vi "AOL Control-4ch_AC.vi"() -> ()   [LabVIEW 2020]
uses:
  TypeDef/Frequency-4ch.ctl
  TypeDef/Amplitude-4ch.ctl
  Globals/FPGA Globals.vi
  <vilib>/DAQmx/create/channels.llb/DAQmx Create Channel (CO-Pulse Generation-Time).vi
  <vilib>/FPGAPlugInAG/PXIe-7976R/niLvFpga_Open_PXIe-7976R.vi
  <vilib>/rvi/interface/common/dynamic/niFpgaDynamicAddResources.vi
  <vilib>/Utility/error.llb/Error Cluster From Error Code.vi
  <vilib>/rvi/errors/niLvFpgaAdjustHostInterfaceError.vi
  <vilib>/FPGAPlugInAG/Dynamic/niLvFpga_Close_Dynamic.vi
  <vilib>/rvi/interface/nirviOpenFPGA/nirviOpenFPGA.xnode
  FPGA Bitfiles/aolcontrolprojec_FPGATarget_Gentrigpulse_Cnv+VIMB-cw_AC.lvbitx
  <vilib>/rvi/interface/nirviReadWriteControl/nirviReadWriteControl.xnode
  <vilib>/rvi/interface/nirviCloseFPGA/nirviCloseFPGA.xnode
  NiFpgaLv.dll
  <vilib>/rvi/interface/Simulation/niFpgaSimulationCallBeginRW.vi
panel:
  in  "Tab Control":T1(tab)
  in  "Use RF from file":bool
  in  "RF Code File":path=path "D:/Microscope data/2019-04-16/Sameer/Packets"
  in  "Frequency (MHz)":T2={"Ch 1"=39, "Ch 2"=39, "Ch 3"=39, "Ch 4"=39} {"Ch 4" min=20 max=50 step=1; "Ch 3" min=20 max=50 step=1; "Ch 2" min=20 max=50 step=1; "Ch 1" min=20 max=50 step=1}
  in  "Amplitude":T3={"Ch 1"=255, "Ch 2"=255, "Ch 3"=255, "Ch 4"=255} {"Ch 4" max=255 step=1; "Ch 3" max=255 step=1; "Ch 2" max=255 step=1; "Ch 1" max=255 step=1}
  in  "Stop":bool
  in  "Load":bool
  in  "Run":bool
  in  "Clear":bool
  in  "Settings":bool
  out "Ethernet Port Opened":bool
  out "RF Loaded":bool
  out "Trigger Sent":bool
  out "Status":string
  in  "Use FlexRIO Trigger":bool=TRUE
  in  "DAQmx Trigger Channel":tag="PXI1Slot4/ctr0"
  in  "Pulse Width (sec)":dbl=1e-05
  in  "Initial Delay(sec)":dbl=0.01 format="%.6f"
  out "Select Device 1":i32=1 caption="Device 1 Port" min=1 max=5 step=1
  out "Select Device 2":i32=1 caption="Device 2 Port" min=1 max=5 step=1
  out "Packet Array":string[](array[string])
  out "No of Packets":i32
  out "FPGA MAC 1":string caption="Device 1 MAC Address"
  out "FPGA MAC 2":string caption="Device 2 MAC Address"
  out "Trigger Error":errorcluster
  in  "error in":errorcluster
  # "User needs to send a single TTL rising edge for the controller to generate RF."
  # "Trigger"
  # "Ethernet"
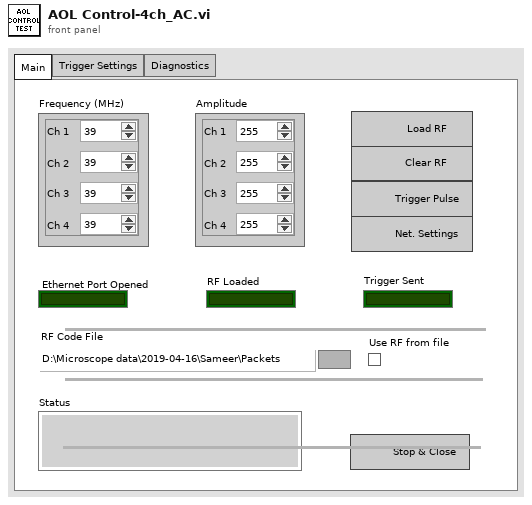
[diagram p1: front panel]
types:
  T1 = enum32{"Main", "Trigger Settings", "Diagnostics"}
  T2 = typedef "Frequency-4ch.ctl" = cluster{"Ch 1":u16, "Ch 2":u16, "Ch 3":u16, "Ch 4":u16}
  T3 = typedef "Amplitude-4ch.ctl" = cluster{"Ch 1":u16, "Ch 2":u16, "Ch 3":u16, "Ch 4":u16}
  T4 = enum8{"Enabled", "Disabled", "Disabled and Grayed Out"}
  T5 = typedef "FPGA Settings.ctl" = cluster{"System Clock(MHz)":dbl, "FPGA MAC 1":string, "Port Number 1":i32, "Port Number 2":i32, "FPGA MAC 2":string, "PC MAC Address":string}
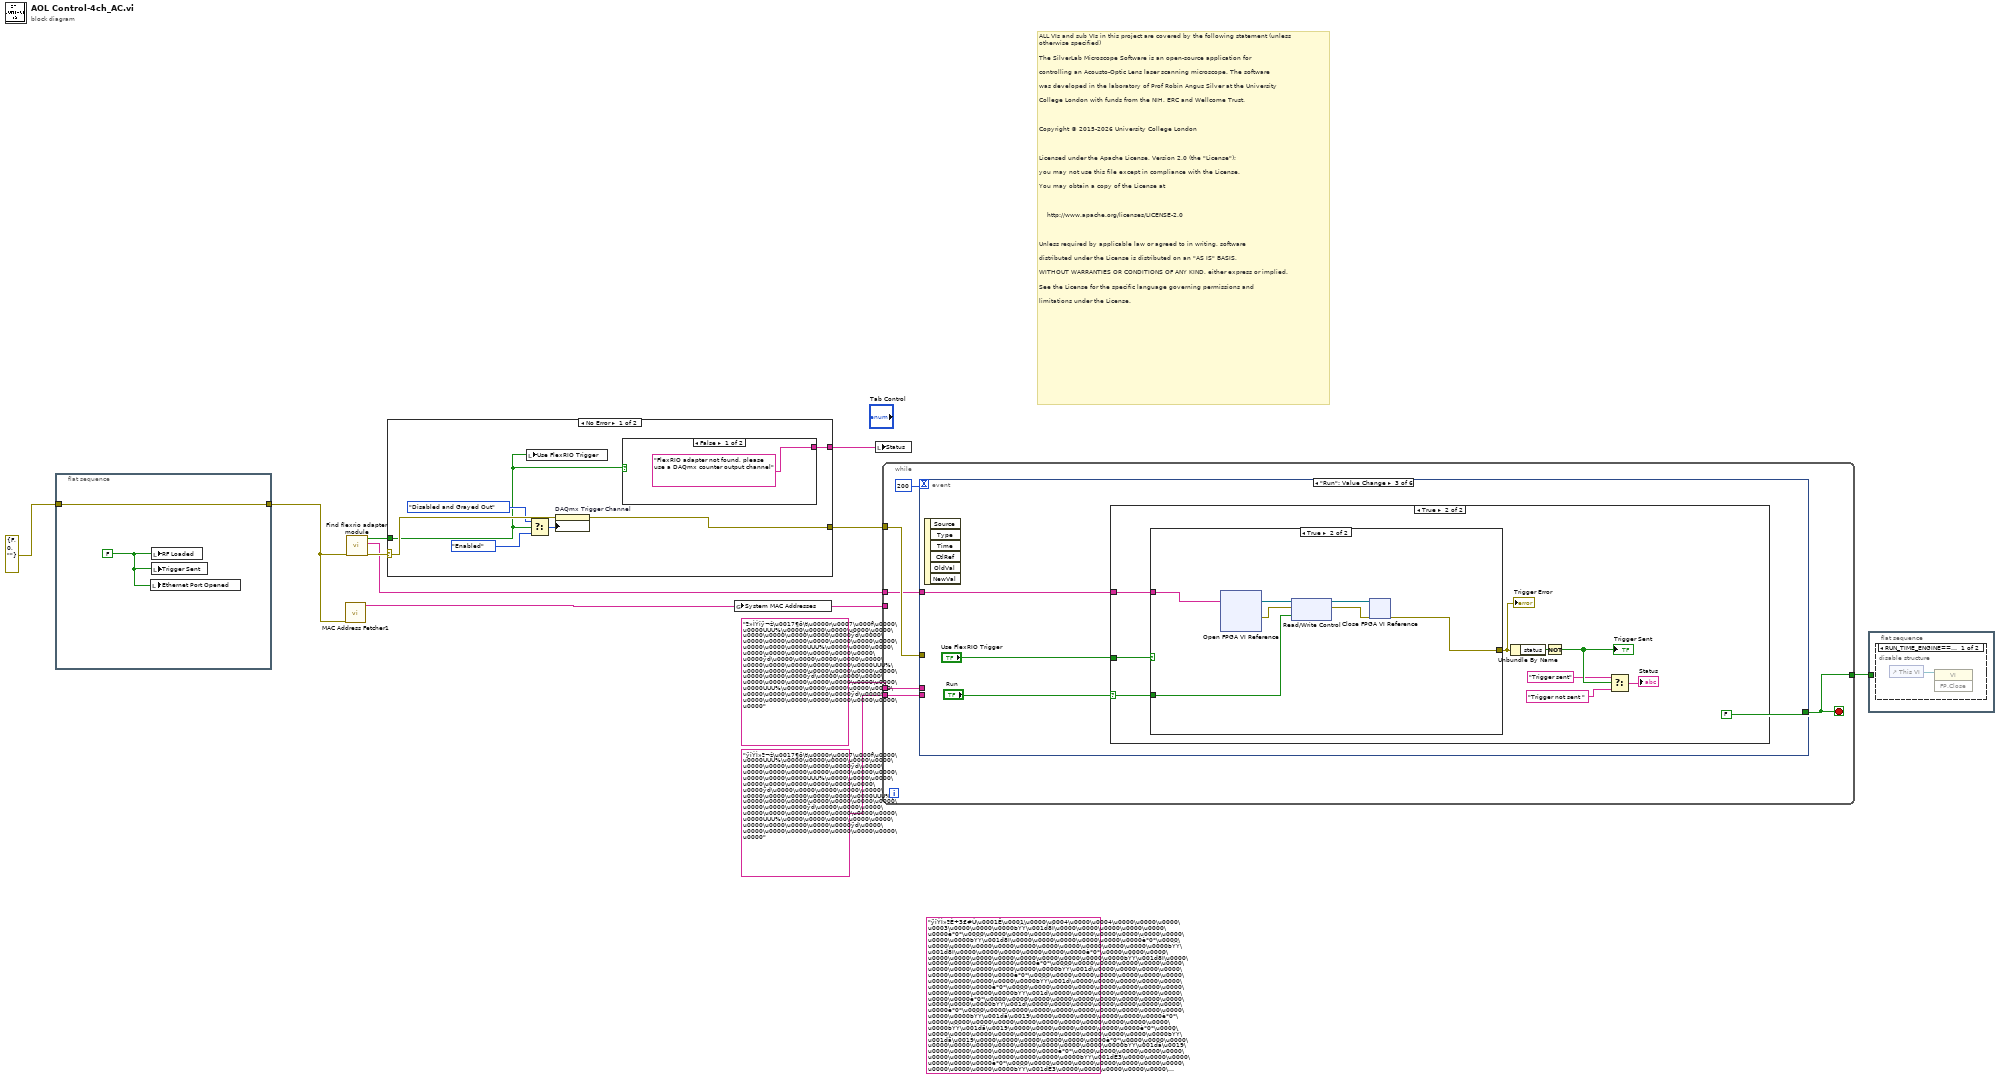
[diagram p0: block diagram]
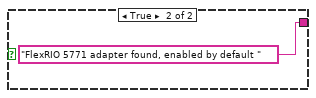
[diagram p2: hidden frame]
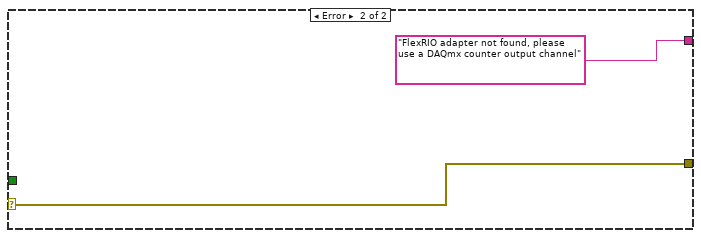
[diagram p3: hidden frame]
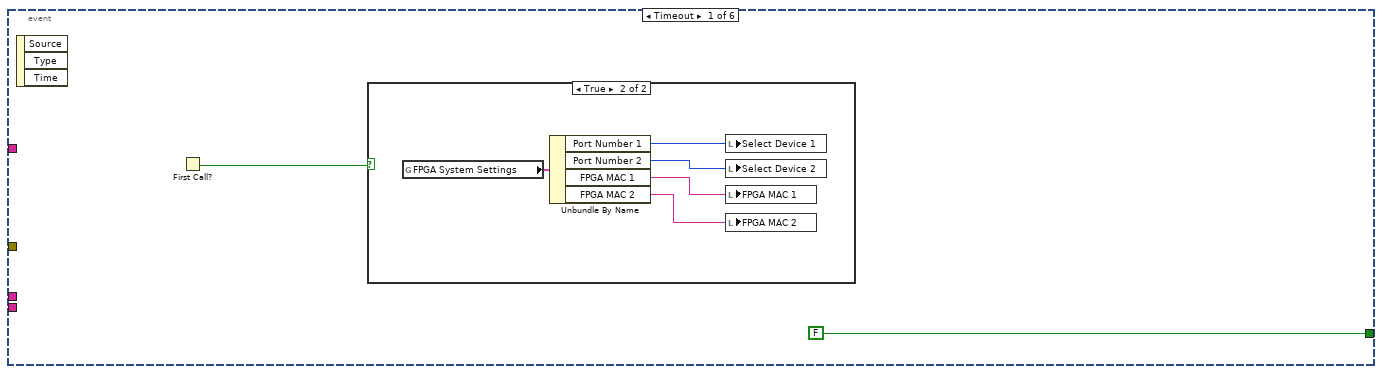
[diagram p5: hidden frame]
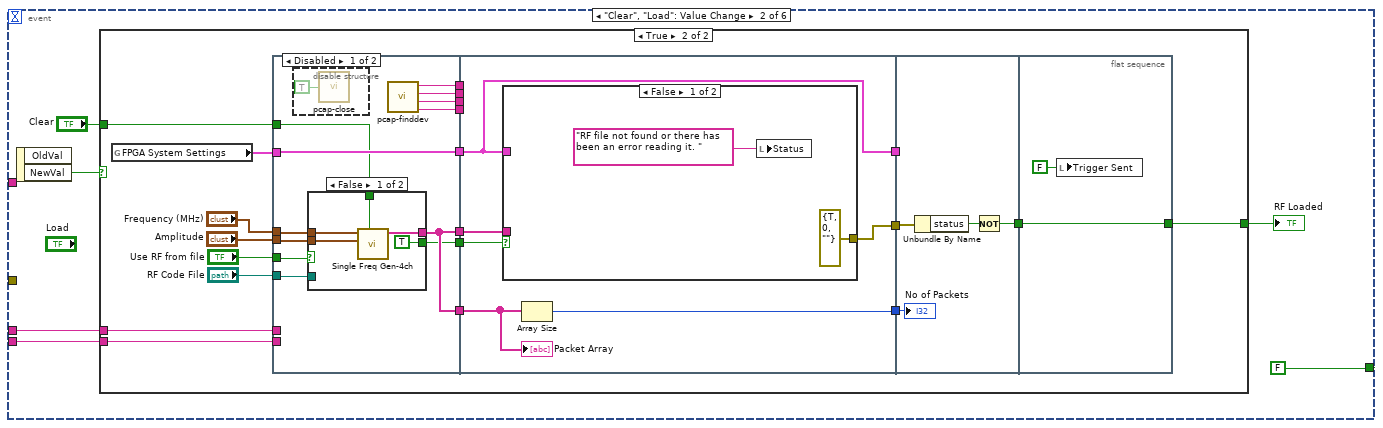
[diagram p7: hidden frame]
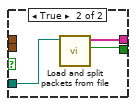
[diagram p9: hidden frame]
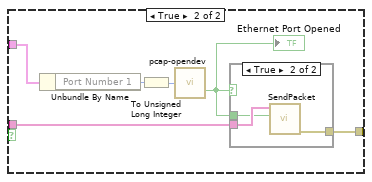
[diagram p11: hidden frame]
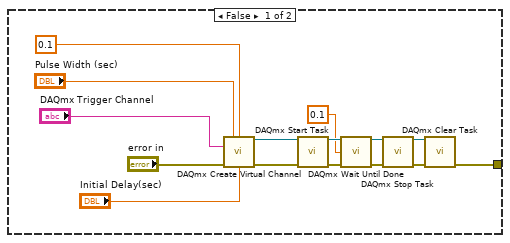
[diagram p14: hidden frame]
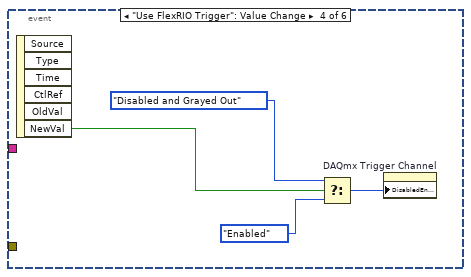
[diagram p15: hidden frame]
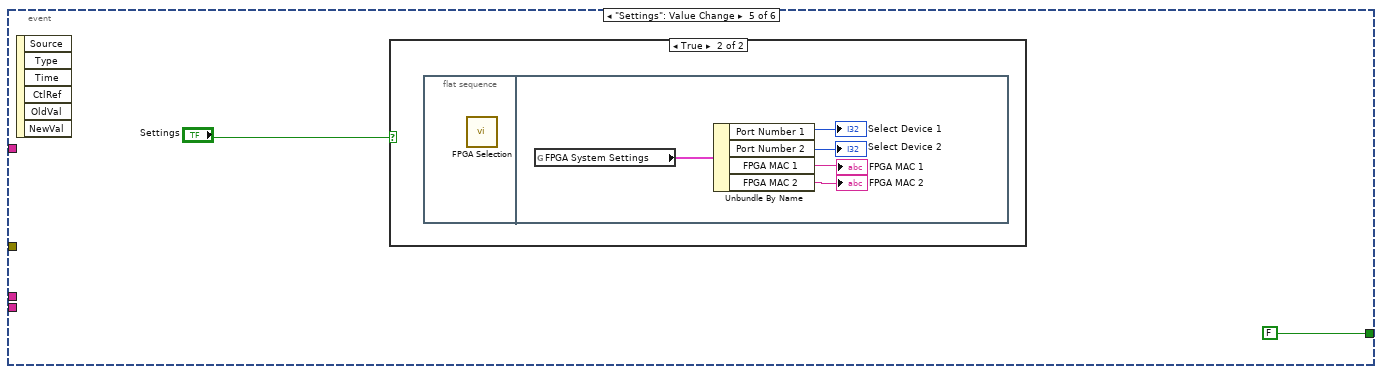
[diagram p16: hidden frame]
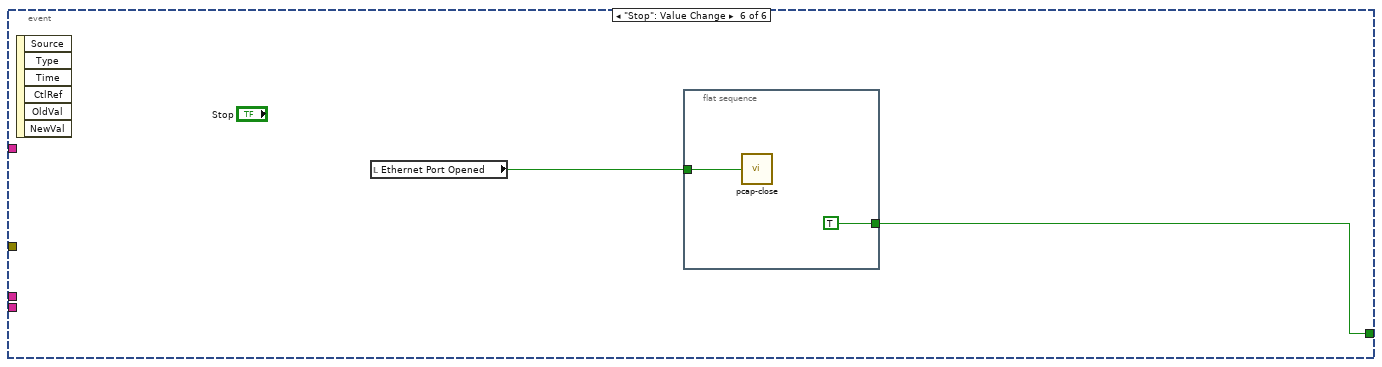
[diagram p18: hidden frame]
diagram:
  (unwired) "ÿîÝÌ»ªÈ÷3£#Ù\u0001Ê\u0001\u0000\u0004\u0000\u0004\u0000\u0000\u0000\u0003\u0000\u0000\u0000ÞÝÝ\u001d8Ì\u0000\u0000\u0000\u0000\u0000\u0000è*0*\u0000\u0000\u0000\u0000\u0000\u0000\u0000\u0000\u0000\u0000\u0000\u0000ÞÝÝ\u001d8Ì\u0000\u0000\u0000\u0000\u0000\u0000è*0*\u0000\u0000\u0000\u0000\u0000\u0000\u0000\u0000\u0000\u0000\u0000\u0000ÞÝÝ\u001d8Ì\u0000\u0000\u0000\u0000\u0000\u0000è*0*\u0000\u0000\u0000\u0000\u0000\u0000\u0000\u0000\u0000\u0000\u0000\u0000ÞÝÝ\u001d8Ì\u0000\u0000\u0000\u0000\u0000\u0000è*0*\u0000\u0000\u0000\u0000\u0000\u0000\u0000\u0000\u0000\u0000\u0000\u0000ÞÝÝ\u001d\u0000\u0000\u0000\u0000\u0000\u0000\u0000\u0000è*0*\u0000\u0000\u0000\u0000\u0000\u0000\u0000\u0000\u0000\u0000\u0000\u0000ÞÝÝ\u001d\u0000\u0000\u0000\u0000\u0000\u0000\u0000\u0000è*0*\u0000\u0000\u0000\u0000\u0000\u0000\u0000\u0000\u0000\u0000\u0000\u0000ÞÝÝ\u001d\u0000\u0000\u0000\u0000\u0000\u0000\u0000\u0000è*0*\u0000\u0000\u0000\u0000\u0000\u0000\u0000\u0000\u0000\u0000\u0000\u0000ÞÝÝ\u001d\u0000\u0000\u0000\u0000\u0000\u0000\u0000\u0000è*0*\u0000\u0000\u0000\u0000\u0000\u0000\u0000\u0000\u0000\u0000\u0000\u0000ÞÝÝ\u001dä\u0019\u0000\u0000\u0000\u0000\u0000\u0000è*0*\u0000\u0000\u0000\u0000\u0000\u0000\u0000\u0000\u0000\u0000\u0000\u0000ÞÝÝ\u001dä\u0019\u0000\u0000\u0000\u0000\u0000\u0000è*0*\u0000\u0000\u0000\u0000\u0000\u0000\u0000\u0000\u0000\u0000\u0000\u0000ÞÝÝ\u001dä\u0019\u0000\u0000\u0000\u0000\u0000\u0000è*0*\u0000\u0000\u0000\u0000\u0000\u0000\u0000\u0000\u0000\u0000\u0000\u0000ÞÝÝ\u001dä\u0019\u0000\u0000\u0000\u0000\u0000\u0000è*0*\u0000\u0000\u0000\u0000\u0000\u0000\u0000\u0000\u0000\u0000\u0000\u0000ÞÝÝ\u001dÈ3\u0000\u0000\u0000\u0000\u0000\u0000è*0*\u0000\u0000\u0000\u0000\u0000\u0000\u0000\u0000\u0000\u0000\u0000\u0000ÞÝÝ\u001dÈ3\u0000\u0000\u0000\u0000\u0000\u0000è*0*\u0000\u0000\u0000\u0000\u0000\u0000\u0000\u0000\u0000\u0000\u0000\u0000ÞÝÝ\u001dÈ3\u0000\u0000\u0000\u0000\u0000\u0000è*0*\u0000\u0000\u0000\u0000\u0000\u0000\u0000\u0000\u0000\u0000\u0000\u0000ÞÝÝ\u001dÈ3\u0000\u0000\u0000\u0000\u0000\u0000è*0*\u0000\u0000\u0000\u0000\u0000\u0000\u0000\u0000\u0000\u0000"
  # "ALL VIs and sub VIs in this project are covered by the following statement (unless \notherwise specified)\n\nThe SilverLab Microscope Software is an open-source application for\n\ncontrolling an Acousto-Optic Lens laser scanning microscope. The software\n\nwas developed in the laboratory of Prof Robin Angus Silver at the University\n\nCollege London with funds from the NIH, ERC and Wellcome Trust.\n\n \n\nCopyright © 2015-2026 University College London\n\n \n\nLicensed under the Apache License, Version 2.0 (the \"License\");\n\nyou may not use this file except in compliance with the License.\n\nYou may obtain a copy of the License at\n\n \n\n    http://www.apache.org/licenses/LICENSE-2.0\n\n \n\nUnless required by applicable law or agreed to in writing, software\n\ndistributed under the License is distributed on an \"AS IS\" BASIS,\n\nWITHOUT WARRANTIES OR CONDITIONS OF ANY KIND, either express or implied.\n\nSee the License for the specific language governing permissions and\n\nlimitations under the License."
  n1 = flat-sequence {
    tunnel: [w13] -> w1
    tunnel: errorcluster {"status"=FALSE, "code"=0, "source"=""} ("error in (no error)") -> [w13]
    frame #0 {
      w12 = FALSE ("RF Loaded")
      n2 = local write "Ethernet Port Opened"(w12) -> ()
      n3 = local write "RF Loaded"(w12) -> ()
      n4 = local write "Trigger Sent"(w12) -> ()
    }
  }
  n5 = call "MAC Address Fetcher1.vi"("error in (no error)"=w1) -> ("MAC Addresses"=w11:string[])  [unwired: 8 in, 2 out]
  n6 = call "Find flexrio adapter module.vi"("error in (no error)"=w1) -> ("error out"=w7:errorcluster, "Devices & Chassis:Provides Link Name"=w4:string, "NI 5772 adapter present ?"=w5:bool)  [unwired: 8 in]
  n7 = case shown="No Error" w7 {
    selector: w7 -> [w20 w24]
    tunnel: w5 -> [w15 _]
    tunnel: [w16 w24] -> w6
    tunnel: [w14 "FlexRIO adapter not found, please use a DAQmx counter output channel"] -> w3
    frame No Error {
      n8 = local write "Use FlexRIO Trigger"(w15) -> ()
      n9 = Select(t=T4."Disabled and Grayed Out" ("Disabled"), s=w15, f=T4."Enabled") -> (s? t:f=w18:T4)
      n10 = property on="DAQmx Trigger Channel" class="DAQmxName"(error in=w20, "DisabledEnum"=w18) -> (error out=w16:errorcluster)  [unwired: 1 in, 1 out]
      n11 = case shown="False" w15 {
        tunnel: ["FlexRIO adapter not found, please use a DAQmx counter output channel" "FlexRIO 5771 adapter found, enabled by default "] -> w14
        frame False {
        }
        frame True {
        }
      }
    }
    frame Error {
    }
  }
  n12 = global write "FPGA Globals.vi" "System MAC Addresses"(w11) -> ()
  n13 = local write "Status"(w3) -> ()
  n14 = while {
    tunnel: w11 -> [_]
    tunnel: "ª»ÌÝîÿ¬ž\u0017¶ö\t\u0000r\u0007\u000f\u0000\u0000UUU%\u0000\u0000\u0000\u0000\u0000\u0000\u0000\u0000\u0000\u0000ÿd\u0000\u0000\u0000\u0000\u0000\u0000\u0000\u0000\u0000\u0000\u0000UUU%\u0000\u0000\u0000\u0000\u0000\u0000\u0000\u0000\u0000\u0000ÿd\u0000\u0000\u0000\u0000\u0000\u0000\u0000\u0000\u0000\u0000\u0000UUU%\u0000\u0000\u0000\u0000\u0000\u0000\u0000\u0000\u0000\u0000ÿd\u0000\u0000\u0000\u0000\u0000\u0000\u0000\u0000\u0000\u0000\u0000UUU%\u0000\u0000\u0000\u0000\u0000\u0000\u0000\u0000\u0000\u0000ÿd\u0000\u0000\u0000\u0000\u0000\u0000\u0000\u0000\u0000" ("String") -> [w29]
    tunnel: "ÿîÝÌ»ª¬ž\u0017¶ö\t\u0000r\u0007\u000f\u0000\u0000UUU%\u0000\u0000\u0000\u0000\u0000\u0000\u0000\u0000\u0000\u0000ÿd\u0000\u0000\u0000\u0000\u0000\u0000\u0000\u0000\u0000\u0000\u0000UUU%\u0000\u0000\u0000\u0000\u0000\u0000\u0000\u0000\u0000\u0000ÿd\u0000\u0000\u0000\u0000\u0000\u0000\u0000\u0000\u0000\u0000\u0000UUU%\u0000\u0000\u0000\u0000\u0000\u0000\u0000\u0000\u0000\u0000ÿd\u0000\u0000\u0000\u0000\u0000\u0000\u0000\u0000\u0000\u0000\u0000UUU%\u0000\u0000\u0000\u0000\u0000\u0000\u0000\u0000\u0000\u0000ÿd\u0000\u0000\u0000\u0000\u0000\u0000\u0000\u0000\u0000" ("String") -> [w28]
    tunnel: [w27] -> w8
    tunnel: w6 -> [w26]
    tunnel: w4 -> [w25]
    stop <- w27 stop-if-true
    n15 = event shown="[2] \"Run\": Value Change" {
      selector: _ -> [_ _ _ _ _ _]
      dyn-events: _ -> [_ _ _ _ _ _]
      timeout: 200 -> [_ _ _ _ _ _]
      tunnel: w29 -> [_ w41 _ _ _ _]
      tunnel: w28 -> [_ w40 _ _ _ _]
      tunnel: [FALSE FALSE FALSE _ FALSE w155] -> w27
      tunnel: w26 -> [_ _ _ _ _ _]
      tunnel: w25 -> [_ _ w109 _ _ _]
      event Timeout {
        n16 = event-data() -> ()  [unwired: 1 in, 3 out]
        n17 = First Call?() -> (First Call?: T/F=w31:bool)
        n18 = case shown="True" w31 {
          frame False {
          }
          frame True {
            n19 = global read "FPGA Globals.vi" "FPGA System Settings"() -> (w37:T5)
            n20 = Unbundle By Name(w37) -> ("Port Number 1"=w36:i32, "Port Number 2"=w35:i32, "FPGA MAC 1"=w34:string, "FPGA MAC 2"=w33:string)
            n21 = local write "Select Device 1"(w36) -> ()
            n22 = local write "Select Device 2"(w35) -> ()
            n23 = local write "FPGA MAC 1"(w34) -> ()
            n24 = local write "FPGA MAC 2"(w33) -> ()
          }
        }
      }
      event "Clear", "Load": Value Change {
        n25 = event-data() -> ("NewVal"=w43:bool)  [unwired: 1 in, 1 out]
        n26 = case shown="True" w43 {
          tunnel: "Clear" -> [_ w57]
          tunnel: w41 -> [_ w52]
          tunnel: w40 -> [_ w51]
          tunnel: [_ w49] -> w38
          frame False {
          }
          frame True {
            n27 = global read "FPGA Globals.vi" "FPGA System Settings"() -> (w58:T5)
            n28 = flat-sequence {
              tunnel: "Amplitude" -> [w76]
              tunnel: "Frequency (MHz)" -> [w75]
              tunnel: [w74] -> w64
              tunnel: w58 -> [w74]
              tunnel: w57 -> [w73]
              tunnel: [w72] -> w56
              tunnel: [w71] -> w55
              tunnel: [w70] -> w54
              tunnel: [w69] -> w53
              tunnel: w52 -> [_]
              tunnel: w51 -> [_]
              tunnel: [w68] -> w50
              tunnel: [w68] -> w47
              tunnel: "Use RF from file" -> [w67]
              tunnel: "RF Code File" -> [w66]
              tunnel: [w65] -> w44
              tunnel: [w91] -> w63
              tunnel: [w90] -> w62
              tunnel: w64 -> [w89]
              tunnel: [w89] -> w61
              tunnel: w56 -> [_]
              tunnel: w55 -> [_]
              tunnel: w54 -> [_]
              tunnel: w53 -> [_]
              tunnel: w50 -> [w88]
              tunnel: w47 -> [w87]
              tunnel: w44 -> [w86]
              tunnel: w63 -> [w105]
              tunnel: w62 -> [w106]
              tunnel: w61 -> [_]
              tunnel: [w103] -> w48
              tunnel: [w108] -> w49
              tunnel: w48 -> [w108]
              frame #0 {
                n29 = disable-structure shown="Disabled" {
                  frame Disabled {
                    n30 = call "pcap-close.vi"("Opened"=TRUE) -> ()
                  }
                  frame Enabled {
                  }
                }
                n31 = case shown="False" w67 {
                  tunnel: w76 -> [w81 _]
                  tunnel: w75 -> [w80 _]
                  tunnel: w73 -> [w79 _]
                  tunnel: [w78 w84] -> w68
                  tunnel: w66 -> [_ w83]
                  tunnel: [TRUE ("OK?") w82] -> w65
                  frame False {
                    n32 = call "Single Freq Gen-4ch.vi"("Stop Single Frquency"=w79, "Amplitude"=w81, "Frequency (MHz)"=w80) -> ("Hex String (Array)"=w78:string[])  [unwired: 7 in, 1 out]
                  }
                  frame True {
                    n33 = call "Load and split packets from file.vi"("Path"=w83) -> ("OK?"=w82:bool, "Hex String"=w84:string[])  [unwired: 7 in, 2 out]
                  }
                }
                n34 = call "pcap-finddev.vi"() -> ("String 4"=w69:string, "String 3"=w70:string, "String 2"=w71:string, "String"=w72:string)  [unwired: 1 in, 1 out]
              }
              frame #1 {
                n35 = case shown="False" w86 {
                  tunnel: [errorcluster {"status"=TRUE, "code"=0, "source"=""} ("error out") w99] -> w91
                  tunnel: w89 -> [_ w96]
                  tunnel: w88 -> [_ w94]
                  frame False {
                    n36 = local write "Status"("RF file not found or there has been an error reading it. " ("Status")) -> ()
                  }
                  frame True {
                    n37 = Unbundle By Name(w96) -> ("Port Number 1"=w98:i32)
                    n38 = To Unsigned Long Integer(number=w98) -> (unsigned 32bit integer=w97:u32)
                    n39 = call "pcap-opendev.vi"("Select Device"=w97) -> ("Opened"=w95:bool)  [unwired: 2 out]
                    "Ethernet Port Opened" <- w95
                    n40 = case shown="True" w95 {
                      tunnel: [_ w102] -> w99
                      tunnel: w94 -> [_ w101]
                      tunnel: w95 -> [_ w100]
                      frame False {
                      }
                      frame True {
                        n41 = call "SendPacket.vi"("Ethernet Port Opened ?"=w100, "Packet Array"=w101) -> ("error out"=w102:errorcluster)  [unwired: 8 in, 1 out]
                      }
                    }
                  }
                }
                n42 = Array Size(array=w87) -> (size(s)=w90:i32)
                "Packet Array" <- w87
              }
              frame #2 {
                n43 = Unbundle By Name(w105) -> ("status"=w104:bool)
                n44 = Not(x=w104) -> (.not. x?=w103:bool)
                "No of Packets" <- w106
              }
              frame #3 {
                n45 = local write "Trigger Sent"(FALSE ("Trigger Sent")) -> ()
              }
            }
          }
        }
        "RF Loaded" <- w38
      }
      event "Run": Value Change {
        n46 = event-data() -> ()  [unwired: 1 in, 6 out]
        n47 = case shown="True" "Run" {
          selector: "Run" -> [_ w114]
          tunnel: "Use FlexRIO Trigger" -> [_ w121]
          tunnel: w109 -> [_ w113]
          frame False {
          }
          frame True {
            n48 = case shown="True" w121 {
              tunnel: [w122 w138] -> w120
              tunnel: w114 -> [_ w141]
              tunnel: w113 -> [_ w137]
              frame False {
                n49 = call-poly <vilib>:"DAQmx Create Virtual Channel.vi"("high time"="Pulse Width (sec)", "low time"=0.1 ("Pulse Low Time(sec)"), "counter"="DAQmx Trigger Channel", "error in"="error in", "initial delay"="Initial Delay(sec)") -> ("task out"=w131:refnum<k21>, "error out"=w130:errorcluster)  [unwired: 9 in]
                n50 = call <vilib>:"DAQmx Start Task.vi"("task/channels in"=w131, "error in"=w130) -> ("task out"=w129:refnum<k21>, "error out"=w125:errorcluster)  [unwired: 12 in]
                n51 = call <vilib>:"DAQmx Wait Until Done.vi"("task/channels in"=w129, "timeout (sec)"=0.1, "error in"=w125) -> ("task out"=w124:refnum<k21>, "error out"=w123:errorcluster)  [unwired: 11 in]
                n52 = call <vilib>:"DAQmx Stop Task.vi"("task/channels in"=w124, "error in"=w123) -> ("task out"=w128:refnum<k21>, "error out"=w127:errorcluster)  [unwired: 12 in]
                n53 = call <vilib>:"DAQmx Clear Task.vi"("task in"=w128, "error in"=w127) -> ("error out"=w122:errorcluster)  [unwired: 13 in]
              }
              frame True {
                n54 = xnode "Open FPGA VI Reference"("resource name"=w137) -> ("FPGA VI Reference Out"=w143:refnum<k20>, "error out"=w142:errorcluster)  [unwired: 1 in]
                n55 = xnode "Read/Write Control"("FPGA VI Reference In"=w143, "error in"=w142, "TL Input"=w141) -> ("FPGA VI Reference Out"=w140:refnum<k20>, "error out"=w139:errorcluster)
                n56 = xnode "Close FPGA VI Reference"("FPGA VI Reference In"=w140, "error in"=w139) -> ("error out"=w138:errorcluster)
              }
            }
            "Trigger Error" <- w120
            n57 = Unbundle By Name(w120) -> ("status"=w119:bool)
            n58 = Not(x=w119) -> (.not. x?=w118:bool)
            "Trigger Sent" <- w118
            n59 = Select(t="Trigger sent", s=w118, f="Trigger not sent ") -> (s? t:f=→"Status":string)
          }
        }
      }
      event "Use FlexRIO Trigger": Value Change {
        n60 = event-data() -> ("NewVal"=w147:bool)  [unwired: 1 in, 5 out]
        n61 = Select(t=T4."Disabled and Grayed Out" ("Disabled"), s=w147, f=T4."Enabled" ("Disabled")) -> (s? t:f=w144:T4)
        n62 = property on="DAQmx Trigger Channel" class="DAQmxName"("DisabledEnum"=w144) -> ()  [unwired: 2 in, 2 out]
      }
      event "Settings": Value Change {
        n63 = event-data() -> ()  [unwired: 1 in, 6 out]
        n64 = case shown="True" "Settings" {
          frame False {
          }
          frame True {
            n65 = flat-sequence {
              frame #0 {
                n66 = call "FPGA Selection.vi"() -> ()  [unwired: 12 in]
              }
              frame #1 {
                n67 = global read "FPGA Globals.vi" "FPGA System Settings"() -> (w152:T5)
                n68 = Unbundle By Name(w152) -> ("Port Number 1"=→"Select Device 1":i32, "Port Number 2"=→"Select Device 2":i32, "FPGA MAC 1"=→"FPGA MAC 1":string, "FPGA MAC 2"=→"FPGA MAC 2":string)
              }
            }
          }
        }
      }
      event "Stop": Value Change {
        n69 = event-data() -> ()  [unwired: 1 in, 6 out]
        n70 = local read "Ethernet Port Opened"() -> (w156:bool)
        n71 = flat-sequence {
          tunnel: w156 -> [w158]
          tunnel: [TRUE] -> w155
          frame #0 {
            n72 = call "pcap-close.vi"("Opened"=w158) -> ()
          }
        }
      }
    }
  }
  n73 = flat-sequence {
    tunnel: w8 -> [_]
    frame #0 {
      n74 = disable-structure shown="RUN_TIME_ENGINE==True" {
        frame condition #0 {
          n75 = control-ref of="This VI"() -> (w159:refnum<vi>)
          n76 = invoke class="VI" method="FP.Close"(reference=w159) -> ()  [unwired: 2 in, 3 out]
        }
        frame condition #1 (active) {
        }
      }
    }
  }
